vi "generate comb.vi"(4 "maxY":dbl=1.0, 5 "Name Visible":bool, 6 "minY":dbl, 7 "Plot Ref":refnum<vi>, 8 "freq array":dbl[](array[numeric]), 11 "plot list IN":cluster{dbl[], dbl[]}[](array[cluster])) -> (3 "plot list OUT":cluster{dbl[], dbl[]}[](array[cluster]))   [LabVIEW 2021]
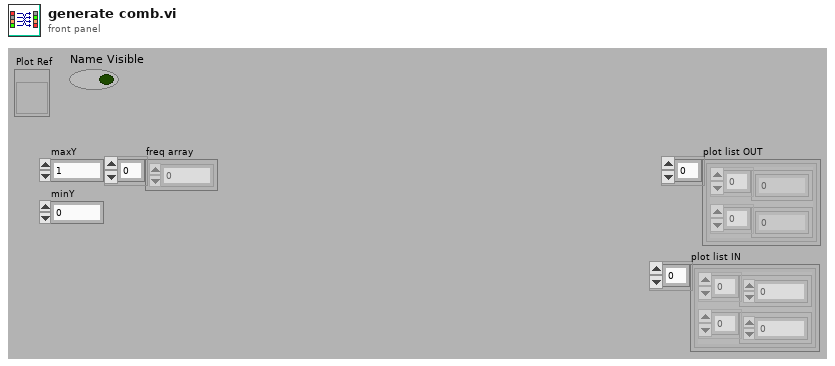
[diagram p1: front panel]
types:
  T1 = cluster{"Name":string, "Color":u32, "Style":u8, "Point Style":u8, "Name Visible":bool, "Allow Drag":bool, "Annotation Mode":u32, "Plot":i32, "Index":i32, "Position":cluster{"X":dbl, "Y":dbl}, "X Scale":u32, "Y Scale":u32, "Show Arrow":bool, "Lock Name":bool, "Plot Area":i32, "Label Offset":cluster{"X":dbl, "Y":dbl}}
  T2 = typedef "LVAnnotationListTypeDef.ctl" = cluster{"Name":string, "Color":u32, "Style":u8, "Point Style":u8, "Name Visible":bool, "Allow Drag":bool, "Annotation Mode":u32, "Plot":i32, "Index":i32, "Position":cluster{"X":dbl, "Y":dbl}, "X Scale":u32, "Y Scale":u32, "Show Arrow":bool, "Lock Name":bool, "Plot Area":i32, "Label Offset":cluster{"X":dbl, "Y":dbl}}[]
  T3 = typedef "LVRangeTypeDef.ctl" = cluster{"Minimum":dbl, "Maximum":dbl, "Increment":dbl, "Minor Increment":dbl, "Start":dbl}
  T4 = cluster{"Name":string, "Color":u32, "Style":u8, "Point Style":u8, "Name Visible":bool, "Allow Drag":bool, "Annotation Mode":u32, "Plot":i32, "Index":i32, "Position":cluster{"X":dbl, "Y":dbl}, "X Scale":u32, "Y Scale":u32, "Show Arrow":bool, "Lock Name":bool, "Plot Area":i32, "Label Offset":cluster{"X":dbl, "Y":dbl}}[]
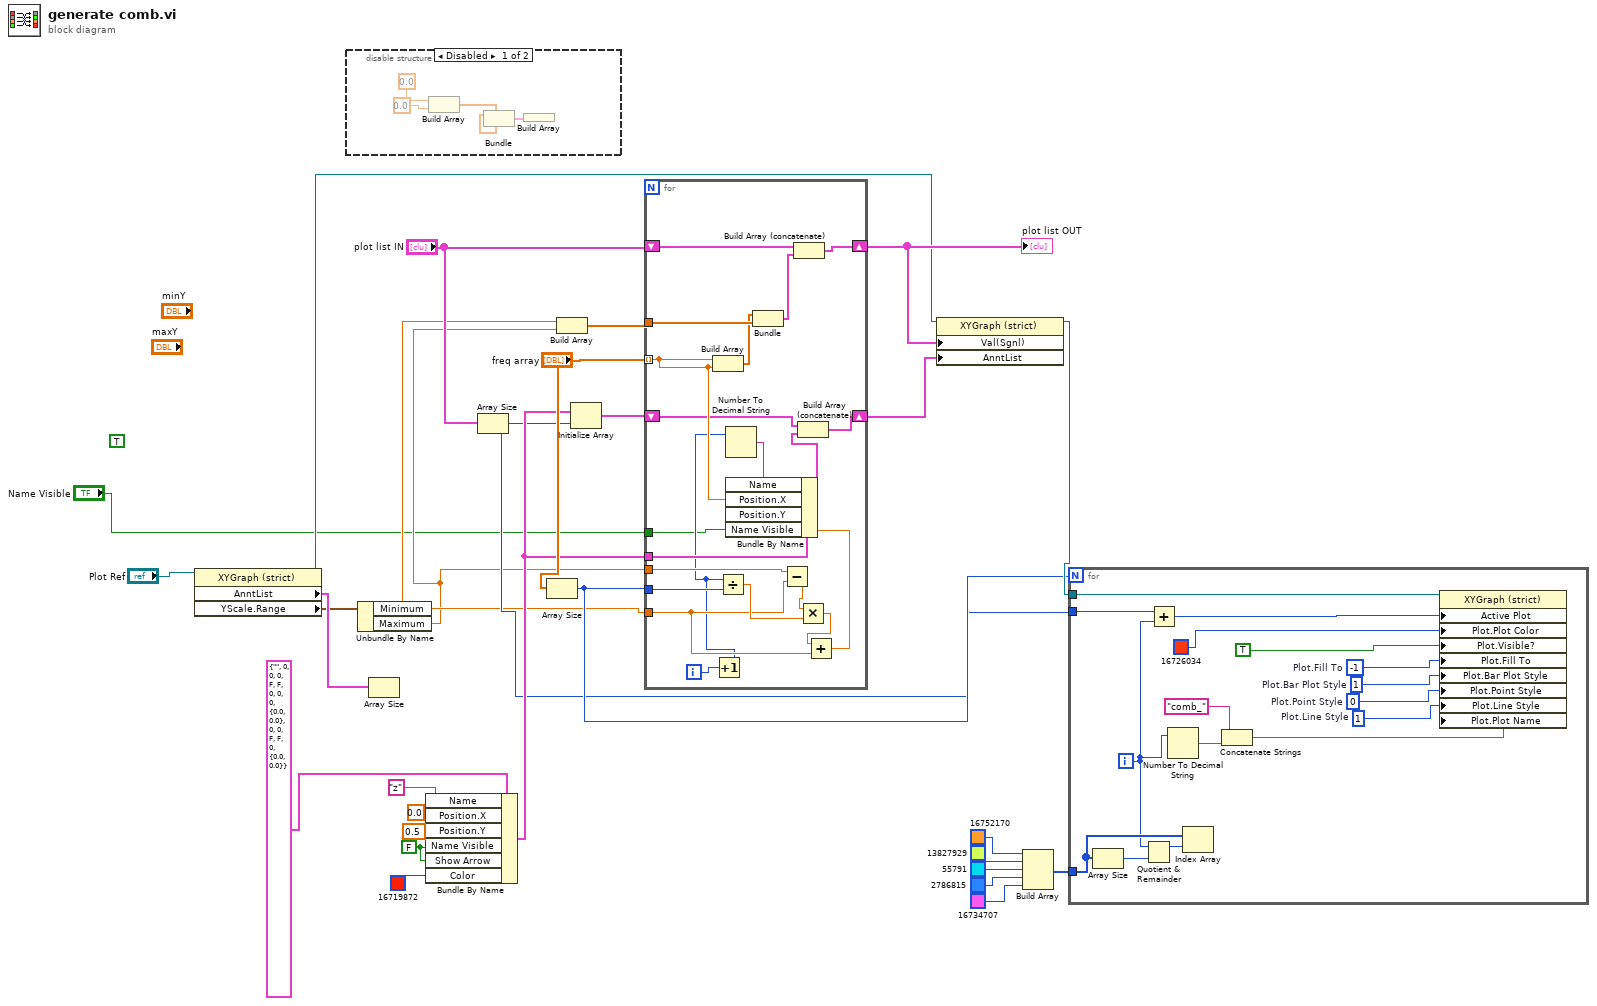
[diagram p0: block diagram]
diagram:
  (unwired) TRUE ("Name Visible")
  w24 = FALSE ("Name Visible")
  n1 = property class="XYGraph (strict)"(reference="Plot Ref") -> (reference out=w10:refnum<vi>, "AnntList"=w9:T2, "YScale.Range"=w4:T3)  [unwired: 1 in, 1 out]
  n2 = disable-structure shown="Disabled" {
    frame Disabled {
      n3 = Build Array(0.0 ("element"), 0.0 ("element")) -> (w31:dbl[])
      n4 = Bundle(w31) -> (w30:cluster{dbl[], void})  [unwired: 2 in]
      n5 = Build Array(w30) -> ()  [unwired: 1 out]
    }
    frame Enabled {
    }
  }
  n6 = Unbundle By Name(w4) -> ("Minimum"=w3:dbl, "Maximum"=w2:dbl)
  n7 = Array Size(array=w9) -> ()  [unwired: 1 out]
  n8 = Bundle By Name(cluster=T1 {"Name"="", "Color"=0, "Style"=0, "Point Style"=0, "Name Visible"=FALSE, "Allow Drag"=FALSE, "Annotation Mode"=0, "Plot"=0, "Index"=0, "Position"={"X"=0.0, "Y"=0.0}, "X Scale"=0, "Y Scale"=0, "Show Arrow"=FALSE, "Lock Name"=FALSE, "Plot Area"=0, "Label Offset"={"X"=0.0, "Y"=0.0}} ("element 2"), "Name"="z", "Position.X"=0.0, "Position.Y"=0.5, "Name Visible"=w24, "Show Arrow"=w24, "Color"=u32 16719872) -> (w8:T1)
  n9 = Array Size(array="plot list IN") -> (size(s)=w5:i32)
  n10 = Array Size(array="freq array") -> (size(s)=w6:i32)
  n11 = Build Array(w3, w2) -> (w29:dbl[])
  n12 = Initialize Array(w8, w5) -> (w7:T4)
  n13 = for {
    shift-right: [w53] -> w12
    shift-left: "plot list IN" -> [w54]
    tunnel: w29 -> [w51]
    tunnel: "freq array" -> [w46] mode=indexing
    shift-right: [w49] -> w13
    shift-left: w7 -> [w44]
    tunnel: w8 -> [w48]
    tunnel: w6 -> [w43]
    tunnel: w2 -> [w42]
    tunnel: w3 -> [w38]
    tunnel: "Name Visible" -> [w34]
    i -> [w36]
    n14 = Build Array(w46, w46) -> (w50:dbl[])
    n15 = Increment(x=w36) -> (x+1=w35:i32)
    n16 = Divide(x=w35, y=w43) -> (x/y=w40:dbl)
    n17 = Number To Decimal String(number=w35) -> (decimal integer string=w47:string)  [unwired: 1 in]
    n18 = Bundle(w50, w51) -> (w52:cluster{dbl[], dbl[]})  [unwired: 1 in]
    n19 = Subtract(x=w42, y=w38) -> (x-y=w41:dbl)
    n20 = Build Array (concatenate)(w54, w52) -> (w53:cluster{dbl[], dbl[]}[])
    n21 = Multiply(x=w41, y=w40) -> (x*y=w39:dbl)
    n22 = Add(x=w39, y=w38) -> (x+y=w37:dbl)
    n23 = Bundle By Name(cluster=w48, "Name"=w47, "Position.X"=w46, "Position.Y"=w37, "Name Visible"=w34) -> (w45:T1)
    n24 = Build Array (concatenate)(w44, w45) -> (w49:T4)
  }
  "plot list OUT" <- w12
  n25 = property on="Property Node" class="XYGraph (strict)"(reference=w10, "Val(Sgnl)"=w12, "AnntList"=w13) -> (reference out=w15:refnum<vi>)  [unwired: 1 in, 1 out]
  n26 = Build Array(u32 16752170, u32 13827929, u32 55791, u32 2786815, u32 16734707) -> (w16:u32[])
  n27 = for {
    N: w6 -> [_]
    tunnel: w16 -> [w64]
    tunnel: w15 -> [w63]
    tunnel: w5 -> [w59]
    i -> [w58]
    w62 = u8 1  # Plot.Line Style
    w65 = u8 0  # Plot.Point Style
    w66 = u8 1  # Plot.Bar Plot Style
    w67 = i16 -1  # Plot.Fill To
    n28 = Array Size(array=w64) -> (size(s)=w69:i32)
    n29 = Quotient & Remainder(x=w58, y=w69) -> (x-y*floor(x/y)=w68:i32)  [unwired: 1 out]
    n30 = Add(x=w59, y=w58) -> (x+y=w70:i32)
    n31 = Number To Decimal String(number=w58) -> (decimal integer string=w57:string)  [unwired: 1 in]
    n32 = Index Array(array=w64, index=w68) -> ()  [unwired: 1 out]
    n33 = Concatenate Strings("comb_", w57) -> (w55:string)
    n34 = property on="Property Node" class="XYGraph (strict)"(reference=w63, "Active Plot"=w70, "Plot.Plot Color"=u32 16726034, "Plot.Visible?"=TRUE ("Plot.Visible"), "Plot.Fill To"=w67, "Plot.Bar Plot Style"=w66, "Plot.Point Style"=w65, "Plot.Line Style"=w62, "Plot.Plot Name"=w55) -> ()  [unwired: 1 in, 2 out]
  }
